vi "Config-Write Key (path).vi"(0 "configuration file path":path, 2 "section":string="General", 7 "key":string="CFTS Run Mode", 9 "value":path, 11 "error in (no error)":errorcluster) -> (4 "file path":path, 8 "found?":bool, 15 "error out":errorcluster)   [LabVIEW 2020]
uses:
  <vilib>/Utility/config.llb/Write Key (Path).vi
  <vilib>/Utility/config.llb/NI_LVConfig.lvlib
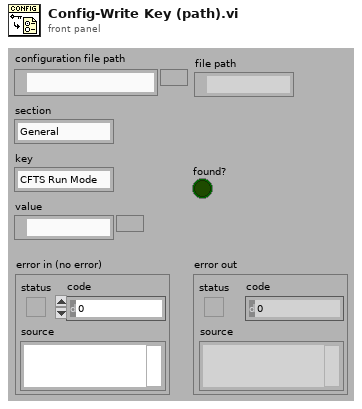
[diagram p1: front panel]
types:
  T1 = typedef "NI_LVConfig.lvlib/Config Data RefNum.ctl" = refnum<k1>
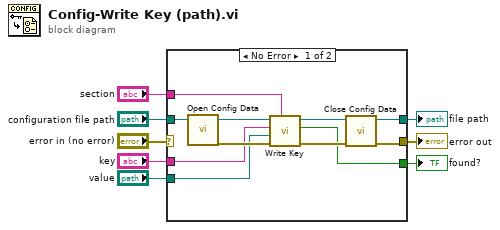
[diagram p0: block diagram]
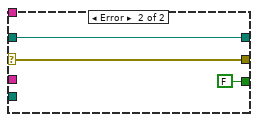
[diagram p2: hidden frame]
diagram:
  n1 = case shown="No Error" "error in (no error)" {
    selector: "error in (no error)" -> [_ w22]
    tunnel: [w17 w22] -> w8
    tunnel: "value" -> [w14 _]
    tunnel: "key" -> [w13 _]
    tunnel: "section" -> [w12 _]
    tunnel: "configuration file path" -> [w11 w21]
    tunnel: [w10 w21] -> w2
    tunnel: [w9 FALSE ("found?")] -> w1
    frame No Error {
      n2 = call <vilib>:"Open Config Data.vi"("configuration file path"=w11) -> ("error out"=w19:errorcluster, "refnum"=w18:T1)  [unwired: 8 in, 1 out]
      n3 = call-poly <vilib>:"Write Key.vi"("section"=w12, "error in (no error)"=w19, "value"=w14, "key"=w13, "refnum"=w18) -> ("error out"=w16:errorcluster, "found?"=w9:bool, "refnum out"=w15:T1)  [unwired: 4 in]
      n4 = call <vilib>:"Close Config Data.vi"("error in (no error)"=w16, "refnum"=w15) -> ("error out"=w17:errorcluster, "file path"=w10:path)  [unwired: 8 in]
    }
    frame Error {
    }
  }
  "error out" <- w8
  "file path" <- w2
  "found?" <- w1
